vi "Initialize Master.vi"(8 "error in":errorcluster, 11 "Serial Master in":refnum<class "Serial Master.lvclass">) -> (0 "error out":errorcluster, 3 "Serial Master out":refnum<class "Serial Master.lvclass">)   [LabVIEW 2012, in "Serial Master.lvclass"]
doc: "This provides an interface for the master to open a connection to the slave."
uses:
  Serial Master.lvclass
  Serial Master.lvclass/Serial Master.ctl
  Transmission Data Unit/Serial Interface/Serial Data Unit.lvclass
  Read VISA resource name.vi
  Read Serial Data Unit.vi
  Read Baud Rate.vi
  Read Parity.vi
  Read Flow Control.vi
  Serial Shared Components/Serial Shared Components.lvlib
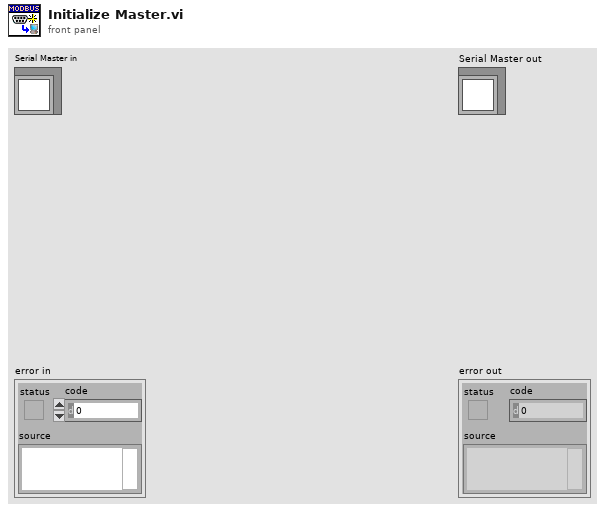
[diagram p1: front panel]
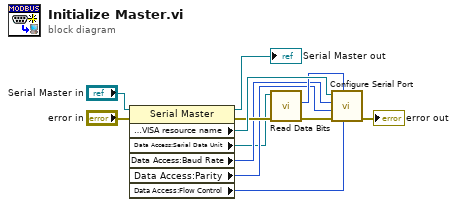
[diagram p0: block diagram]
diagram:
  n1 = property class="Serial Master"(reference="Serial Master in", error in="error in") -> (reference out=→"Serial Master out":refnum<class "Serial Master.lvclass">, error out=w10:errorcluster, "Data Access:VISA resource name"=w11:refnum<visa-resource-name>, "Data Access:Serial Data Unit"=w1:refnum<class "Serial Data Unit.lvclass">, "Data Access:Baud Rate"=w7:u32, "Data Access:Parity"=w6:u16, "Data Access:Flow Control"=w5:u16)
  n2 = call-dynamic "Read Data Bits.vi"("error in (no error)"=w10, "Serial Data Unit in"=w1) -> ("error out"=w9:errorcluster, "data bits"=w8:u16)  [unwired: 7 in, 1 out]
  n3 = call "Configure Serial Port.vi"("Flow Control"=w5, "data bits"=w8, "error in (no error)"=w9, "Parity"=w6, "Baud Rate"=w7, "VISA Refnum in"=w11) -> ("error out"=→"error out":errorcluster)  [unwired: 5 in]
